vi "Initialize.vi"(8 "error in (no error)":errorcluster, 10 "VI Filepath":path) -> (0 "error out":errorcluster, 3 "UI_Interaction_Manager out":refnum<class "UI_Interaction_Manager.lvclass">)   [LabVIEW 2011, in "UI_Interaction_Manager.lvclass"]
uses:
  UI_Interaction_Manager.lvclass
  UI_Interaction_Manager.lvclass/UI_Interaction_Manager.ctl
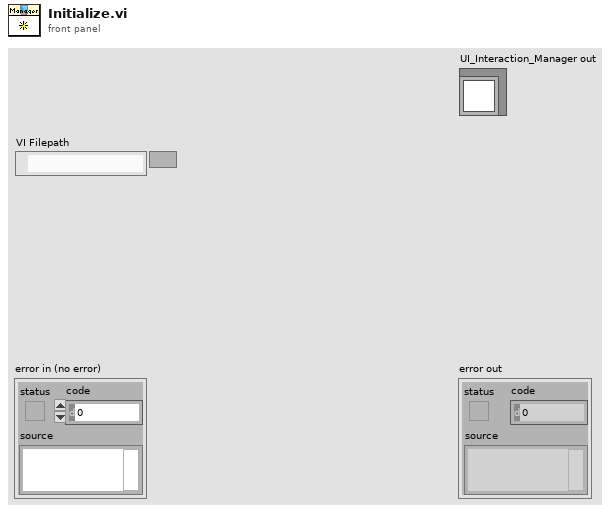
[diagram p1: front panel]
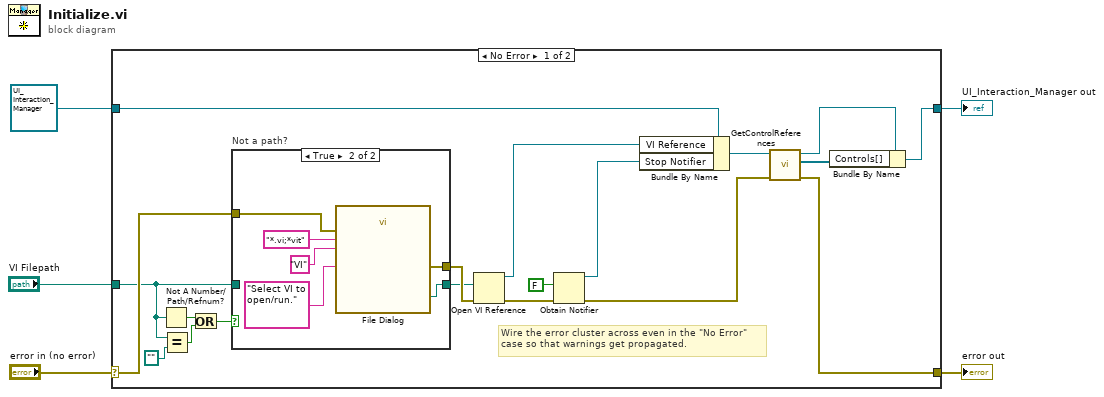
[diagram p0: block diagram]
diagram:
  n1 = case shown="No Error" "error in (no error)" {
    selector: "error in (no error)" -> [w13 w34]
    tunnel: [w14 w34] -> w4
    tunnel: [w16 w33] -> w3
    tunnel: refnum<class "UI_Interaction_Manager.lvclass"> refnum ("UI_Interaction_Manager in") -> [w22 w33]
    tunnel: "VI Filepath" -> [w7 _]
    frame No Error {
      # "Wire the error cluster across even in the \"No Error\"\ncase so that warnings get propagated."
      n2 = Not A Number/Path/Refnum?(number/path/refnum=w7) -> (NaN/Path/Refnum?=w9:bool)
      n3 = Equal?(x=w7, y=path "") -> (x = y?=w8:bool)
      n4 = Or(x=w9, y=w8) -> (x .or. y?=w10:bool)
      n5 = case "Not a path?" shown="True" w10 {
        tunnel: w7 -> [w26 _]
        tunnel: w13 -> [w25 w29]
        tunnel: [w25 w28] -> w12
        tunnel: [w26 w27] -> w11
        frame False {
          # "Valid path."
        }
        frame True {
          n6 = call "File Dialog"("prompt"="Select VI to open/run.", "error in"=w29, "pattern (all files)"="*.vi;*vit", "pattern label"="VI") -> ("selected path"=w27:path, "error out"=w28:errorcluster)  [unwired: 8 in, 2 out]
        }
      }
      n7 = Open VI Reference(vi path=w11, error in (no error)=w12) -> (vi reference=w21:refnum<vi>, error out=w24:errorcluster)  [unwired: 4 in]
      n8 = Obtain Notifier(notification data type=FALSE, error in (no error)=w24) -> (notifier out=w20:refnum<notifier>, error out=w19:errorcluster)  [unwired: 2 in, 1 out]
      n9 = Bundle By Name(cluster=w22, "VI Reference"=w21, "Stop Notifier"=w20) -> (w17:refnum<class "UI_Interaction_Manager.lvclass">)
      n10 = call "GetControlReferences.vi"("error in (no error)"=w19, "UI_Interaction_Manager in"=w17) -> ("error out"=w14:errorcluster, "Controls[] out"=w18:refnum<vi>[], "UI_Interaction_Manager out"=w15:refnum<class "UI_Interaction_Manager.lvclass">)  [unwired: 7 in]
      n11 = Bundle By Name(cluster=w15, "Controls[]"=w18) -> (w16:refnum<class "UI_Interaction_Manager.lvclass">)
    }
    frame Error {
    }
  }
  "error out" <- w4
  "UI_Interaction_Manager out" <- w3
